vi "testFPGA.vi"() -> ()   [LabVIEW 2016]
uses:
  <vilib>/rvi/Emulation/niFpgaGetClockAttributes.vi
  <vilib>/rvi/Emulation/niFpgaSctlEmulationGetInTimedLoop.vi
  <vilib>/rvi/Emulation/niFpgaEmulationReportErrorSimple.vi
  <vilib>/rvi/eio/common/nirviEmuTemplateMethod_errors.vi
  <vilib>/rvi/Emulation/niFpgaCriticalErrorInLSC.vi
  <vilib>/eio/EIOMethodNode/EIOMethodNode.xnode
panel:
  in  "MotorsON":bool=TRUE
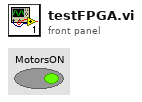
[diagram p1: front panel]
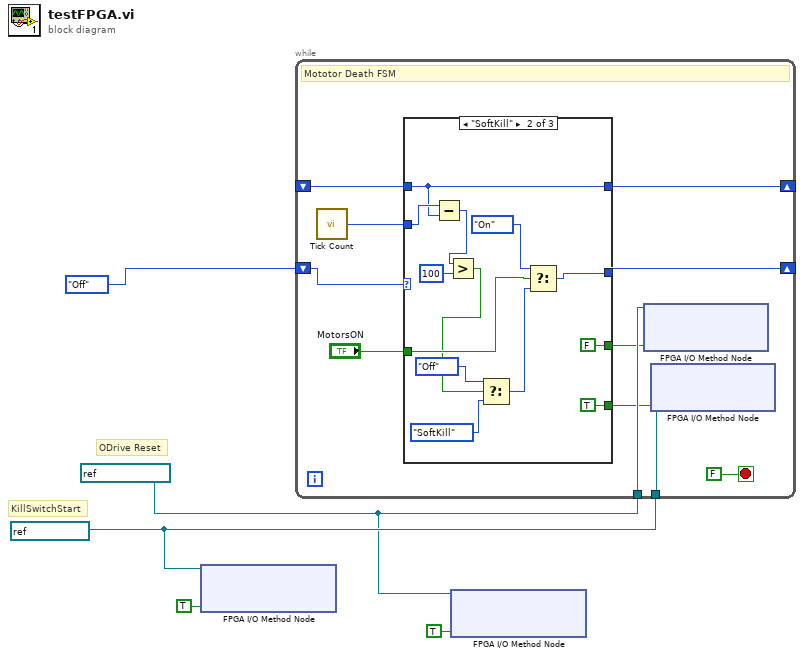
[diagram p0: block diagram]
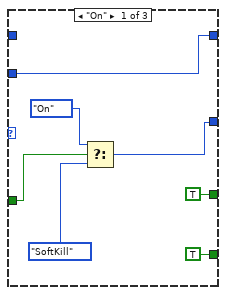
[diagram p2: hidden frame]
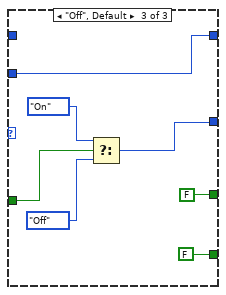
[diagram p3: hidden frame]
diagram:
  w4 = refnum<k21> "DIO/DIO0" ("Transmit")
  w3 = refnum<k21> "MXP/DIO13" ("Transmit")
  # "KillSwitchStart"
  # "ODrive Reset"
  n1 = xnode "FPGA I/O Method Node"("FPGA I/O In"=w4, "Enable"=TRUE) -> ()  [unwired: 1 out]
  n2 = while {
    shift-right: [w6] -> _
    shift-left: enum16{"On", "SoftKill", "Off"}."Off" -> [w15]
    shift-right: [w14] -> _
    shift-left: _ -> [w12]
    tunnel: w3 -> [w11]
    tunnel: w4 -> [w10]
    stop <- FALSE stop-if-true
    # "Mototor Death FSM"
    n3 = call "Tick Count"() -> ("Tick Count(mSec)"=w13:u16)
    n4 = case shown="\"SoftKill\"" w15 {
      tunnel: [w23 w24 w43] -> w14
      tunnel: w13 -> [w23 w25 w43]
      tunnel: w12 -> [_ w24 _]
      tunnel: [TRUE FALSE FALSE] -> w9
      tunnel: [TRUE TRUE FALSE] -> w8
      tunnel: "MotorsON" -> [w20 w34 w40]
      tunnel: [w17 w32 w37] -> w6
      frame "On" {
        n5 = Select(t=enum16{"On", "SoftKill", "Off"}."On", s=w20, f=enum16{"On", "SoftKill", "Off"}."SoftKill") -> (s? t:f=w17:enum16{"On", "SoftKill", "Off"})
      }
      frame "SoftKill" {
        n6 = Subtract(x=w25, y=w24) -> (x-y=w31:u16)
        n7 = Greater?(x=w31, y=u16 100) -> (0:w29:bool)
        n8 = Select(t=enum16{"On", "SoftKill", "Off"}."Off", s=w29, f=enum16{"On", "SoftKill", "Off"}."SoftKill") -> (s? t:f=w26:enum16{"On", "SoftKill", "Off"})
        n9 = Select(t=enum16{"On", "SoftKill", "Off"}."On", s=w34, f=w26) -> (s? t:f=w32:enum16{"On", "SoftKill", "Off"})
      }
      frame "Off", Default {
        n10 = Select(t=enum16{"On", "SoftKill", "Off"}."On", s=w40, f=enum16{"On", "SoftKill", "Off"}."Off") -> (s? t:f=w37:enum16{"On", "SoftKill", "Off"})
      }
    }
    n11 = xnode "FPGA I/O Method Node"("FPGA I/O In"=w11, "Data"=w9) -> ()  [unwired: 1 out]
    n12 = xnode "FPGA I/O Method Node"("FPGA I/O In"=w10, "Data"=w8) -> ()  [unwired: 1 out]
  }
  n13 = xnode "FPGA I/O Method Node"("FPGA I/O In"=w3, "Enable"=TRUE) -> ()  [unwired: 1 out]
